vi "ClimbSequencer.vi"(1 "Master State":enum16{"Normal", "Climb"}(ring)) -> ()   [LabVIEW 2020]
doc: "This VI contains the endgame climb sequencer."
uses:
  sensordata.vi
  drivercommands.vi
  robotoutputs.vi
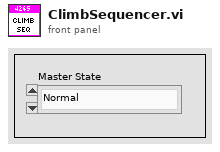
[diagram p1: front panel]
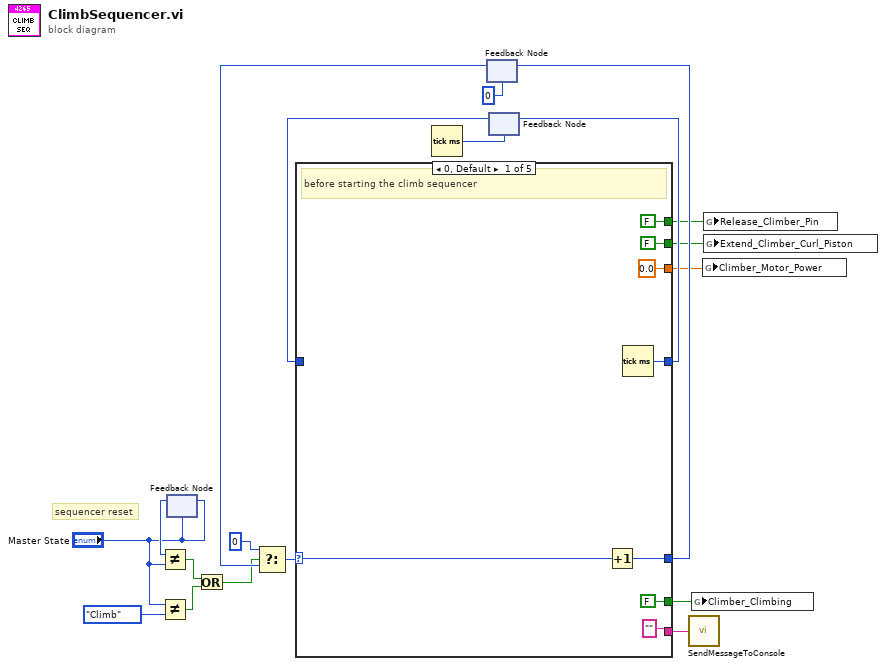
[diagram p0: block diagram]
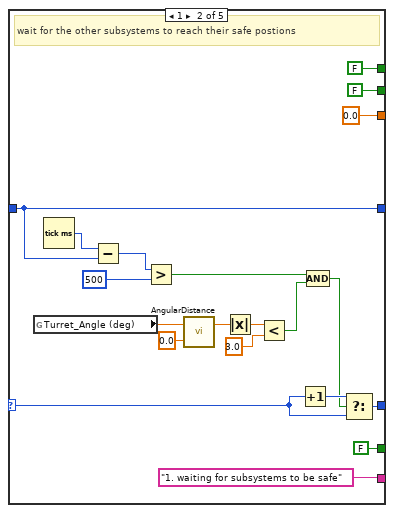
[diagram p2: hidden frame]
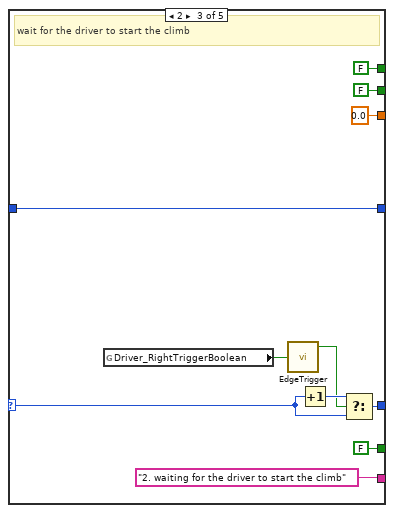
[diagram p3: hidden frame]
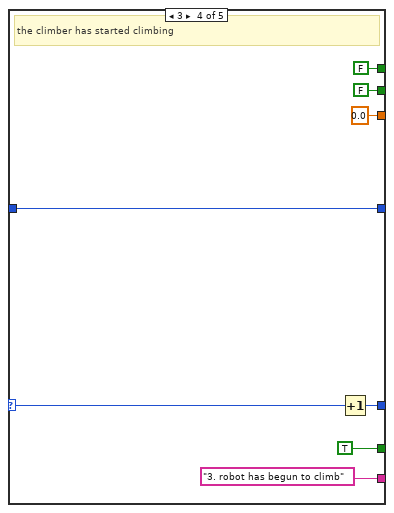
[diagram p4: hidden frame]
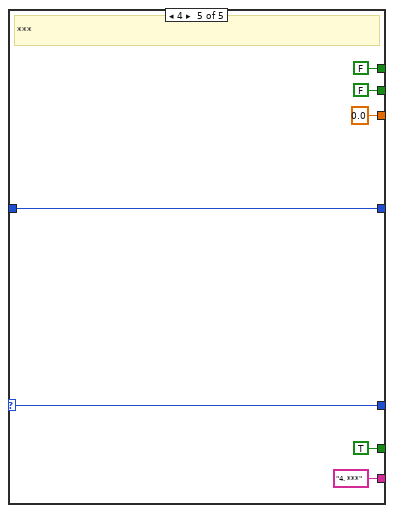
[diagram p5: hidden frame]
diagram:
  # "sequencer reset"
  n1 = Not Equal?(x="Master State", y=enum16{"Normal", "Climb"}."Climb") -> (x != y?=w2:bool)
  n2 = feedback-in #1("Master State") -> ()
  n3 = feedback #1("Master State") -> (w11:enum16{"Normal", "Climb"})
  n4 = Not Equal?(x=w11, y="Master State") -> (x != y?=w5:bool)
  n5 = Or(x=w5, y=w2) -> (x .or. y?=w4:bool)
  n6 = Tick Count (ms)() -> (millisecond timer value=w16:u32)
  n7 = feedback #2(0) -> (w17:i32)
  n8 = Select(t=0, s=w4, f=w17) -> (s? t:f=w19:i32)
  n9 = feedback #3(w16) -> (w15:u32)
  n10 = case shown="0, Default" w19 {
    selector: w19 -> [w25 w45 w58 w66 w72]
    tunnel: [w24 w44 w56 w62 w72] -> w12
    tunnel: ["" "1. waiting for subsystems to be safe" "2. waiting for the driver to start the climb" "3. robot has begun to climb" "4. ***"] -> w10
    tunnel: [w27 w40 w54 w65 w73] -> w14
    tunnel: w15 -> [_ w40 w54 w65 w73]
    tunnel: [FALSE FALSE FALSE TRUE TRUE] -> w9
    tunnel: [FALSE FALSE FALSE FALSE FALSE] -> w8
    tunnel: [FALSE FALSE FALSE FALSE FALSE] -> w7
    tunnel: [0.0 0.0 0.0 0.0 0.0] -> w6
    frame 0, Default {
      # "before starting the climb sequencer"
      n11 = Increment(x=w25) -> (x+1=w24:i32)
      n12 = Tick Count (ms)() -> (millisecond timer value=w27:u32)
    }
    frame 1 {
      # "wait for the other subsystems to reach their safe postions"
      n13 = global read "sensordata.vi" "Turret_Angle (deg)"() -> (w37:dbl)
      n14 = Tick Count (ms)() -> (millisecond timer value=w42:u32)
      n15 = Subtract(x=w42, y=w40) -> (x-y=w43:u32)
      n16 = Greater?(x=w43, y=u32 500) -> (0:w39:bool)
      n17 = call "AngularDistance.vi"("Goal Angle (deg) [0,360]"=0.0, "Current Angle (deg) [-Inf,+Inf]"=w37) -> ("Signed Angular Distance (deg) [-180,+180]"=w35:dbl)  [unwired: 1 out]
      n18 = Absolute Value(x=w35) -> (abs(x)=w34:dbl)
      n19 = Less?(x=w34, y=3.0) -> (x < y?=w32:bool)
      n20 = Increment(x=w45) -> (x+1=w46:i32)
      n21 = Compound Arithmetic op=AND(w39, w32) -> (w38:bool)
      n22 = Select(t=w46, s=w38, f=w45) -> (s? t:f=w44:i32)
    }
    frame 2 {
      # "wait for the driver to start the climb"
      n23 = global read "drivercommands.vi" "Driver_RightTriggerBoolean"() -> (w53:bool)
      n24 = call "EdgeTrigger.vi"("Input Signal"=w53) -> ("Rising Edge Trigger"=w52:bool)  [unwired: 2 out]
      n25 = Increment(x=w58) -> (x+1=w57:i32)
      n26 = Select(t=w57, s=w52, f=w58) -> (s? t:f=w56:i32)
    }
    frame 3 {
      # "the climber has started climbing"
      n27 = Increment(x=w66) -> (x+1=w62:i32)
    }
    frame 4 {
      # "***"
    }
  }
  n28 = feedback-in #2(w12) -> ()
  n29 = feedback-in #3(w14) -> ()
  n30 = call "SendMessageToConsole.vi"("Message String"=w10) -> ()  [unwired: 1 in]
  n31 = global write "robotoutputs.vi" "Climber_Climbing"(w9) -> ()
  n32 = global write "robotoutputs.vi" "Climber_Motor_Power"(w6) -> ()
  n33 = global write "robotoutputs.vi" "Release_Climber_Pin"(w8) -> ()
  n34 = global write "robotoutputs.vi" "Extend_Climber_Curl_Piston"(w7) -> ()
